vi "Generate XML File.vi"(8 "error in (no error)":errorcluster, 10 "Code Coverage":map{path, dbl}(c390), 11 "Coverage Report in":refnum<class "Coverage Report.lvclass">) -> (0 "error out":errorcluster, 2 "Report Path":path, 3 "Coverage Report out":refnum<class "Coverage Report.lvclass">)   [LabVIEW 2020, in "Coverage Report.lvclass"]
uses:
  Coverage Report.lvclass
  Coverage Report.lvclass/Coverage Report.ctl
  <vilib>/xml/Close Reference(Node).vi
  <vilib>/xml/NI_XML.lvlib
  <resource>/objmgr/DOMUserDefRef.rc
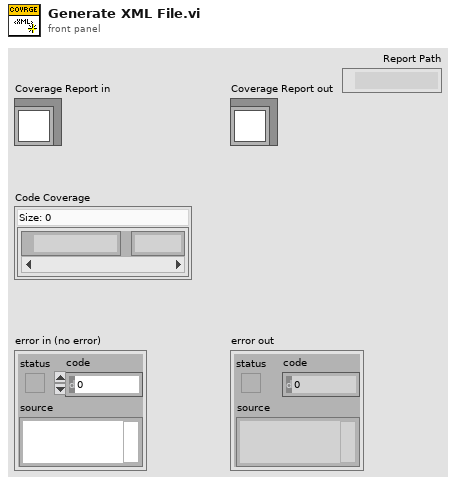
[diagram p1: front panel]
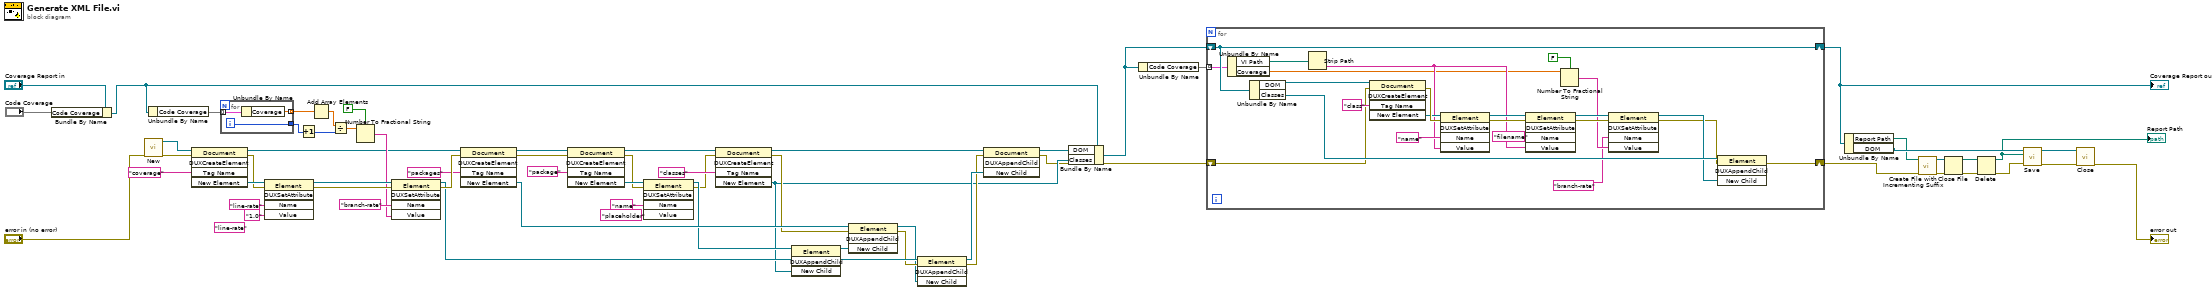
[diagram p0: block diagram]
diagram:
  (unwired) "line-rate" ("Name")
  n1 = Bundle By Name(cluster="Coverage Report in", "Code Coverage"="Code Coverage") -> (w13:refnum<class "Coverage Report.lvclass">)
  n2 = call <vilib>:"New.vi"("error in (no error)"="error in (no error)") -> ("error out"=w62:errorcluster, "DOM document out"=w63:refnum<k20>)  [unwired: 7 in]
  n3 = Unbundle By Name(w13) -> ("Code Coverage"=w12:map{path, dbl})
  n4 = invoke class="Document" method="DUXCreateElement"(reference=w63, error in=w62, "Tag Name"="coverage") -> (reference out=w43:refnum<k20>, error out=w55:errorcluster, "New Element"=w56:refnum<k20>)  [unwired: 2 in, 2 out]
  n5 = for {
    tunnel: w12 -> [w66] mode=indexing
    tunnel: [w65] -> w49 mode=indexing
    tunnel: [w64] -> w47
    i -> [w64]
    n6 = Unbundle By Name(w66) -> ("Coverage"=w65:dbl)
  }
  n7 = invoke class="Element" method="DUXSetAttribute"(reference=w56, error in=w55, "Name"="line-rate", "Value"="1.0") -> (reference out=w52:refnum<k20>, error out=w51:errorcluster)  [unwired: 1 in, 3 out]
  n8 = Increment(x=w47) -> (x+1=w9:i32)
  n9 = Add Array Elements(numeric array=w49) -> (sum=w48:dbl)
  n10 = Divide(x=w48, y=w9) -> (x/y=w46:dbl)
  n11 = Number To Fractional String(use system decimal point (T)=FALSE, number=w46) -> (F-format string=w44:string)  [unwired: 2 in]
  n12 = invoke class="Element" method="DUXSetAttribute"(reference=w52, error in=w51, "Name"="branch-rate", "Value"=w44) -> (reference out=w40:refnum<k20>, error out=w42:errorcluster)  [unwired: 1 in, 3 out]
  n13 = invoke class="Document" method="DUXCreateElement"(reference=w43, error in=w42, "Tag Name"="packages") -> (reference out=w37:refnum<k20>, error out=w35:errorcluster, "New Element"=w30:refnum<k20>)  [unwired: 2 in, 2 out]
  n14 = invoke class="Document" method="DUXCreateElement"(reference=w37, error in=w35, "Tag Name"="package") -> (reference out=w27:refnum<k20>, error out=w32:errorcluster, "New Element"=w33:refnum<k20>)  [unwired: 2 in, 2 out]
  n15 = invoke class="Element" method="DUXSetAttribute"(reference=w33, error in=w32, "Name"="name", "Value"="placeholder") -> (reference out=w24:refnum<k20>, error out=w22:errorcluster)  [unwired: 1 in, 3 out]
  n16 = invoke class="Document" method="DUXCreateElement"(reference=w27, error in=w22, "Tag Name"="classes") -> (reference out=w26:refnum<k20>, error out=w21:errorcluster, "New Element"=w18:refnum<k20>)  [unwired: 2 in, 2 out]
  n17 = invoke class="Element" method="DUXAppendChild"(reference=w24, "New Child"=w18) -> (reference out=w23:refnum<k20>)  [unwired: 2 in, 3 out]
  n18 = invoke class="Element" method="DUXAppendChild"(reference=w30, error in=w21, "New Child"=w23) -> (reference out=w28:refnum<k20>, error out=w29:errorcluster)  [unwired: 1 in, 2 out]
  n19 = invoke class="Element" method="DUXAppendChild"(reference=w40, error in=w29, "New Child"=w28) -> (reference out=w39:refnum<k20>, error out=w38:errorcluster)  [unwired: 1 in, 2 out]
  n20 = invoke class="Document" method="DUXAppendChild"(reference=w26, error in=w38, "New Child"=w39) -> (reference out=w19:refnum<k20>, error out=w17:errorcluster)  [unwired: 1 in, 2 out]
  n21 = Bundle By Name(cluster=w13, "DOM"=w19, "Classes"=w18) -> (w11:refnum<class "Coverage Report.lvclass">)
  n22 = Unbundle By Name(w11) -> ("Code Coverage"=w10:map{path, dbl})
  n23 = for {
    shift-right: [w84] -> w4
    shift-left: w17 -> [w86]
    shift-right: [w83] -> w16
    shift-left: w11 -> [w83]
    tunnel: w10 -> [w82] mode=indexing
    n24 = Unbundle By Name(w82) -> ("VI Path"=w81:path, "Coverage"=w69:dbl)
    n25 = Unbundle By Name(w83) -> ("DOM"=w88:refnum<k20>, "Classes"=w87:refnum<k20>)
    n26 = Strip Path(path=w81) -> (name=w75:string)  [unwired: 1 out]
    n27 = invoke class="Document" method="DUXCreateElement"(reference=w88, error in=w86, "Tag Name"="class") -> (error out=w85:errorcluster, "New Element"=w80:refnum<k20>)  [unwired: 2 in, 3 out]
    n28 = invoke class="Element" method="DUXSetAttribute"(reference=w80, error in=w85, "Name"="name", "Value"=w75) -> (reference out=w78:refnum<k20>, error out=w77:errorcluster)  [unwired: 1 in, 3 out]
    n29 = invoke class="Element" method="DUXSetAttribute"(reference=w78, error in=w77, "Name"="filename", "Value"=w75) -> (reference out=w74:refnum<k20>, error out=w72:errorcluster)  [unwired: 1 in, 3 out]
    n30 = Number To Fractional String(use system decimal point (T)=FALSE, number=w69) -> (F-format string=w68:string)  [unwired: 2 in]
    n31 = invoke class="Element" method="DUXSetAttribute"(reference=w74, error in=w72, "Name"="branch-rate", "Value"=w68) -> (reference out=w73:refnum<k20>, error out=w71:errorcluster)  [unwired: 1 in, 3 out]
    n32 = invoke class="Element" method="DUXAppendChild"(reference=w87, error in=w71, "New Child"=w73) -> (error out=w84:errorcluster)  [unwired: 1 in, 3 out]
  }
  "Coverage Report out" <- w16
  n33 = Unbundle By Name(w16) -> ("Report Path"=w2:path, "DOM"=w20:refnum<k20>)
  n34 = call <vilib>:"Create File with Incrementing Suffix.vi"("error in (no error)"=w4, "file path"=w2) -> ("error out"=w7:errorcluster, "refnum out"=w8:refnum<file>)  [unwired: 7 in, 1 out]
  n35 = Close File(refnum=w8, error in=w7) -> (path=w6:path, error out=w5:errorcluster)
  n36 = Delete(path (use dialog)=w6, error in=w5) -> (deleted path=w1:path, error out=w3:errorcluster)  [unwired: 3 in, 1 out]
  "Report Path" <- w1
  n37 = call <vilib>:"Save.vi"("error in (no error)"=w3, "XML file path"=w1, "DOM document in"=w20) -> ("error out"=w59:errorcluster, "DOM document out"=w60:refnum<k20>)  [unwired: 6 in, 1 out]
  n38 = call-poly <vilib>:"Close.vi"("error in (no error)"=w59, "node"=w60) -> ("error out"=→"error out":errorcluster)  [unwired: 7 in]
